vi "Cyclic Get Joystick.vi"(7 "# Copies (0 = infinite repeat)":u32, 8 "error in (no error)":errorcluster, 11 "Message Enqueuer":refnum<class "Message Enqueuer.lvclass">) -> (0 "error out":errorcluster, 3 "Message Enqueuer out":refnum<class "Message Enqueuer.lvclass">)   [LabVIEW 2020, in "RPI.SenseHat.Actor.lvlib" / "Update Joystick State Msg.lvclass"]
uses:
  Update Joystick State Msg.lvclass
  C:/Program Files (x86)/National Instruments/LabVIEW 2020/vi.lib/ActorFramework/Message/Message.lvclass
  Z:/Code/Git/WC/RPI.SenseHat/src/RPI.SenseHat.Actor/RPI.SenseHat.Actor Messages/Get Joystick State Msg/Update Joystick State Msg.lvclass
  <vilib>/ActorFramework/Message Enqueuer/Message Enqueuer.lvclass
  <vilib>/ActorFramework/Time-Delayed Send Message/Time-Delay Override Options.ctl
panel:
  out "Delivery Notifier":refnum<notifier>
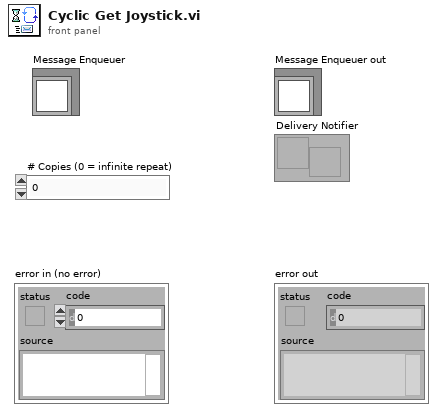
[diagram p1: front panel]
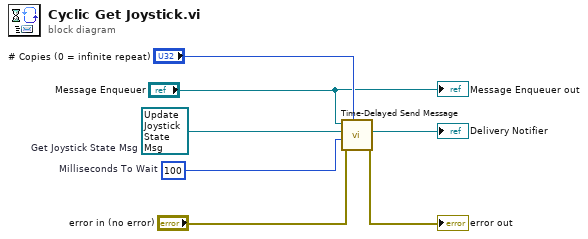
[diagram p0: block diagram]
diagram:
  w6 = 100  # Milliseconds To Wait
  w7 = refnum<class "Update Joystick State Msg.lvclass"> refnum  # Get Joystick State Msg
  n1 = call <vilib>:"Time-Delayed Send Message.vi"("# Copies (0 = infinite repeat)"="# Copies (0 = infinite repeat)", "error in (no error)"="error in (no error)", "Milliseconds To Wait"=w6, "Message"=w7, "Message Enqueuer"="Message Enqueuer") -> ("error out"=→"error out":errorcluster, "Delivery Notifier"=→"Delivery Notifier":refnum<notifier>)  [unwired: 5 in]
  "Message Enqueuer out" <- "Message Enqueuer"
